vi "download_file.vi"(8 "error in (no error)":errorcluster, 10 "target_path":path, 11 "path":string) -> (0 "error out":errorcluster)   [LabVIEW 2015, in "lv-dropbox.lvlib" / "v2.lvlib"]
uses:
  v2.lvlib
  private/_controls/content_type.ctl
  <vilib>/httpClient/POSTBuffer.vi
  private/_subvis/advanced/parse_header-single.vi
  lv-dropbox.lvlib
  <vilib>/httpClient/LabVIEWHTTPClient.lvlib
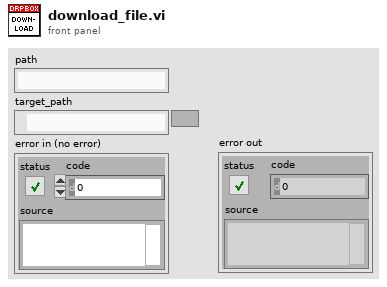
[diagram p1: front panel]
types:
  T1 = typedef "lv-dropbox.lvlib/content_type.ctl" = enum16{"<content_type>", "application/json", "application/octet-stream", "application/x-www-form-urlencoded"}
  T2 = cluster{"name":string, "path_lower":string, "id":string, "client_modified":string, "server_modified":string, "rev":string, "size":u64}
  T3 = enum16{"open", "replace", "create", "open or create", "replace or create", "replace or create with confirmation"}
  T4 = typedef "LabVIEWHTTPClient.lvlib/ClientHandle.ctl" = refnum<k1>
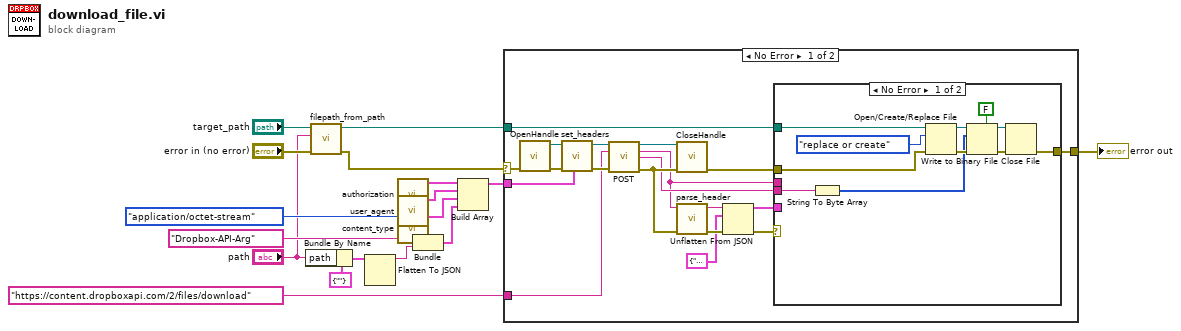
[diagram p0: block diagram]
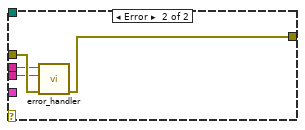
[diagram p2: hidden frame]
diagram:
  n1 = Bundle By Name(cluster=cluster{"path":string} {"path"=""}, "path"="path") -> (w8:cluster{"path":string})
  n2 = call "filepath_from_path.vi"("error in (no error)"="error in (no error)", "path"="path", "filepath in"="target_path") -> ("error out"=w1:errorcluster, "filepath out"=w2:path)  [unwired: 7 in]
  n3 = Flatten To JSON(anything=w8) -> (JSON string=w7:string)  [unwired: 2 in, 1 out]
  n4 = call "authorization.vi"() -> ("header"=w15:cluster{"header":string, "value":string})  [unwired: 11 in]
  n5 = call "user_agent.vi"() -> ("header"=w14:cluster{"header":string, "value":string})  [unwired: 11 in]
  n6 = call "content_type.vi"("content_type"=content_type."application/octet-stream") -> ("header"=w16:cluster{"header":string, "value":string})  [unwired: 10 in]
  n7 = Bundle("header"="Dropbox-API-Arg", "JSON string"=w7) -> (w5:cluster{"header":string, "JSON string":string})  [unwired: 1 in]
  n8 = Build Array(w15, w14, w16, w5) -> (w12:cluster{"header":string, "JSON string":string}[])
  n9 = case shown="No Error" w1 {
    selector: w1 -> [w29 w52]
    tunnel: w12 -> [w18 _]
    tunnel: "https://content.dropboxapi.com/2/files/download" ("url") -> [w28 _]
    tunnel: [w26 w52] -> w10
    tunnel: w2 -> [w20 _]
    frame No Error {
      n10 = call <vilib>:"OpenHandle.vi"("error in (no error)"=w29) -> ("client handle out"=w32:T4, "error out"=w19:errorcluster)  [unwired: 13 in]
      n11 = call "set_headers.vi"("header_value []"=w18, "error in (no error)"=w19, "client_handle in"=w32) -> ("error out"=w30:errorcluster, "client_handle out"=w31:T4)  [unwired: 7 in]
      n12 = call-poly <vilib>:"POST.vi"("client handle"=w31, "url"=w28, "error in (no error)"=w30) -> ("client handle out"=w34:T4, "headers"=w21:string, "body"=w27:string, "error out"=w35:errorcluster)  [unwired: 9 in]
      n13 = call <vilib>:"CloseHandle.vi"("client handle"=w34, "error in (no error)"=w35) -> ("error out"=w23:errorcluster)  [unwired: 13 in]
      n14 = call-poly "parse_header.vi"("error in (no error)"=w35, "headers"=w21) -> ("error out"=w36:errorcluster, "value"=w25:string)  [unwired: 8 in]
      n15 = Unflatten From JSON(JSON string=w25, type and defaults=T2 {"name"="", "path_lower"="", "id"="", "client_modified"="", "server_modified"="", "rev"="", "size"=0}, error in (no error)=w36) -> (value=w22:T2, error out=w24:errorcluster)  [unwired: 4 in]
      n16 = case shown="No Error" w24 {
        tunnel: w27 -> [w42 w49]
        tunnel: [w38 w50] -> w26
        tunnel: w23 -> [w47 w51]
        tunnel: w22 -> [_ _]
        tunnel: w21 -> [_ w48]
        tunnel: w20 -> [w37 _]
        frame No Error {
          n17 = String To Byte Array(string=w42) -> (unsigned byte array=w40:u8[])
          n18 = Open/Create/Replace File(file path (use dialog)=w37, error in=w47, operation (0:open)=T3."replace or create") -> (refnum out=w46:refnum<file>, error out=w43:errorcluster)  [unwired: 3 in, 1 out]
          n19 = Write to Binary File(file (use dialog)=w46, data=w40, error in=w43, 5:FALSE ("prepend array or string size? (T)")) -> (refnum out=w45:refnum<file>, error out=w44:errorcluster)  [unwired: 2 in, 1 out]
          n20 = Close File(refnum=w45, error in=w44) -> (error out=w38:errorcluster)  [unwired: 1 out]
        }
        frame Error {
          n21 = call "error_handler.vi"("error in (no error)"=w51, "body"=w49, "headers"=w48) -> ("error out"=w50:errorcluster)  [unwired: 8 in]
        }
      }
    }
    frame Error {
    }
  }
  "error out" <- w10
